vi "Update Target Value.vi"(11 "Target Info":T1(array[cluster])) -> (3 "Was target seen?":bool)   [LabVIEW 2012]
uses:
  Target Datum.ctl
  Robot Global Data.vi
panel:
  in  "Bottom dividing line":dbl
  in  "Top dividing line":dbl
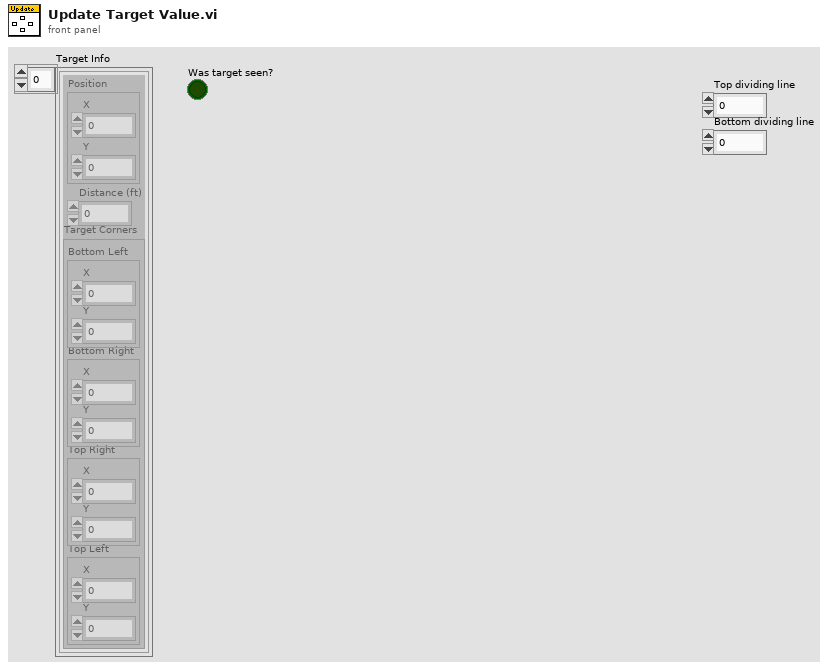
[diagram p1: front panel]
types:
  T1 = cluster{"Position":cluster{"X":dbl, "Y":dbl}, "Distance (ft)":dbl, "Target Corners":cluster{"Bottom Left":cluster{"X":dbl, "Y":dbl}, "Bottom Right":cluster{"X":dbl, "Y":dbl}, "Top Right":cluster{"X":dbl, "Y":dbl}, "Top Left":cluster{"X":dbl, "Y":dbl}}}[]
  T2 = typedef "Target Datum.ctl" = cluster{"Position":cluster{"X":dbl, "Y":dbl}, "Distance (ft)":dbl, "Target Corners":cluster{"Bottom Left":cluster{"X":dbl, "Y":dbl}, "Bottom Right":cluster{"X":dbl, "Y":dbl}, "Top Right":cluster{"X":dbl, "Y":dbl}, "Top Left":cluster{"X":dbl, "Y":dbl}}}
  T3 = cluster{"Left":T2, "Bottom":T2, "Right":T2, "Top":T2}
  T4 = cluster{"Position":cluster{"X":dbl, "Y":dbl}, "Distance (ft)":dbl, "Target Corners":cluster{"Bottom Left":cluster{"X":dbl, "Y":dbl}, "Bottom Right":cluster{"X":dbl, "Y":dbl}, "Top Right":cluster{"X":dbl, "Y":dbl}, "Top Left":cluster{"X":dbl, "Y":dbl}}}
  T5 = typedef "BasketType.ctl" = enum16{"Left", "Bottom", "Right", "Top"}
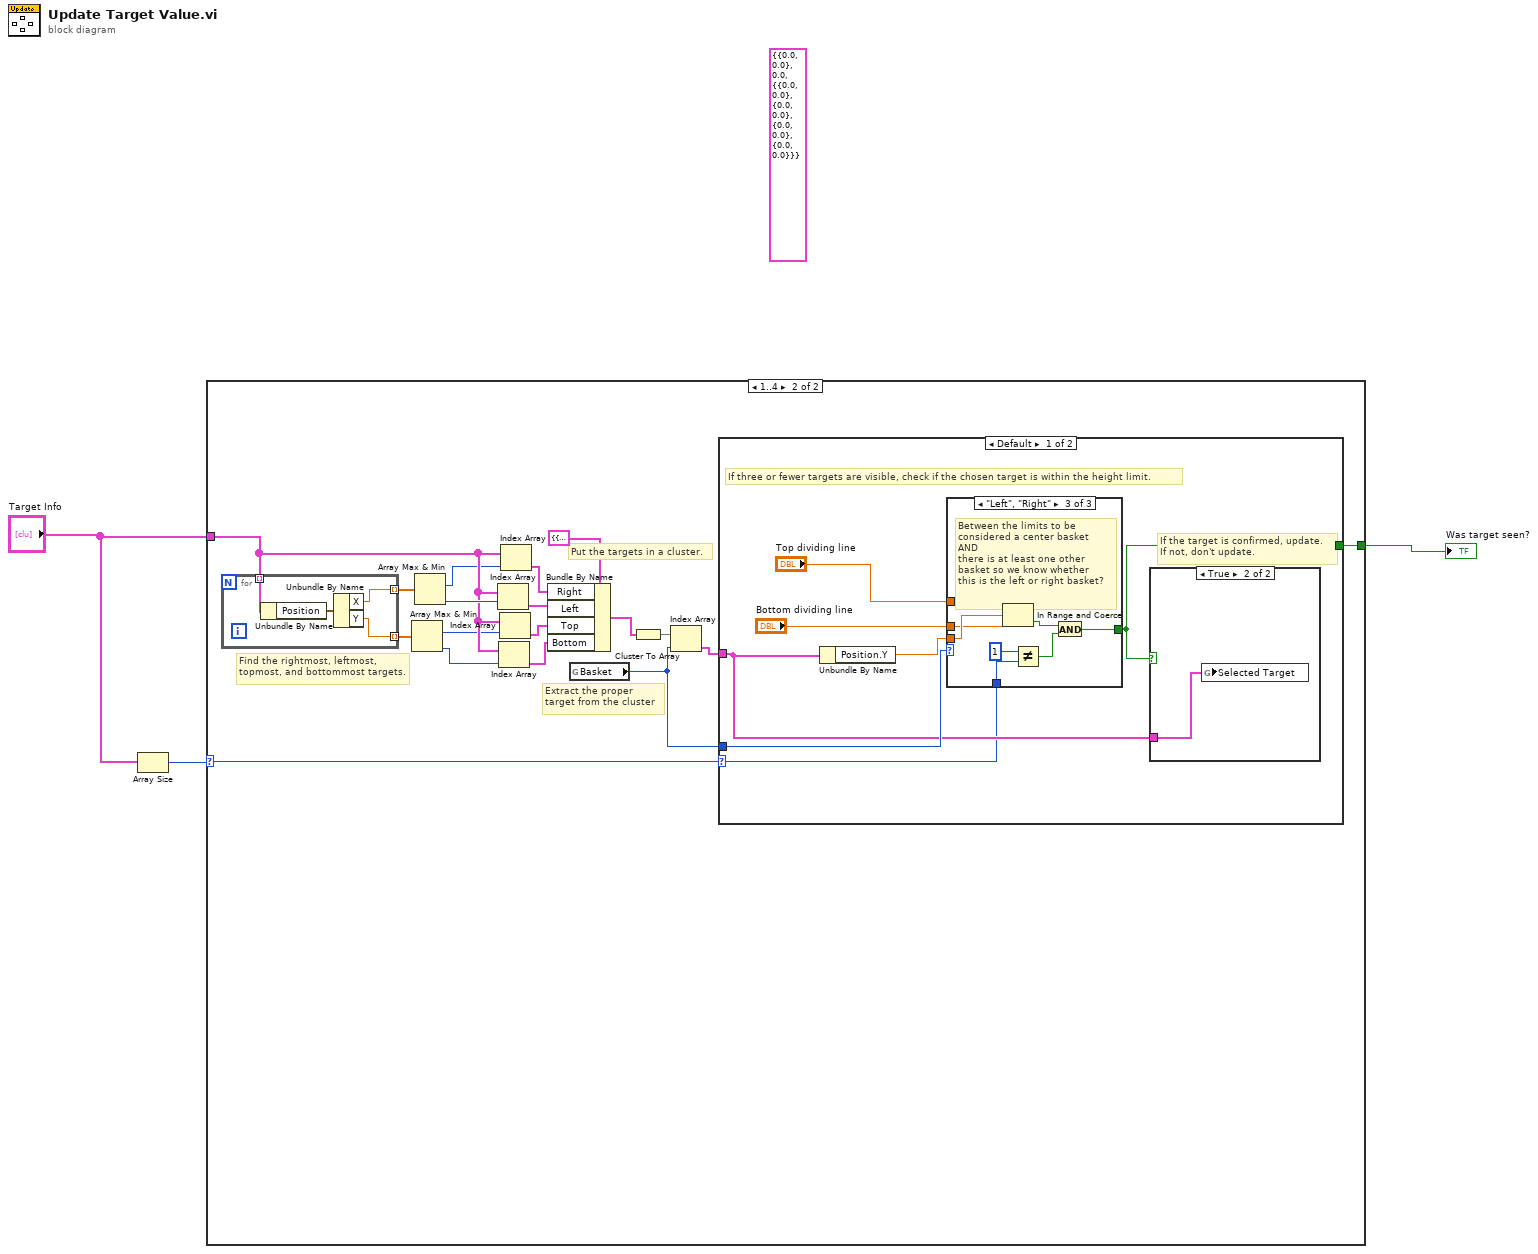
[diagram p0: block diagram]
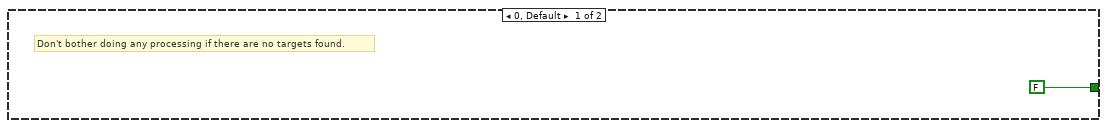
[diagram p2: hidden frame]
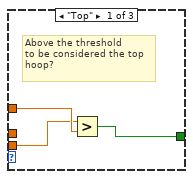
[diagram p4: hidden frame]
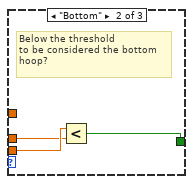
[diagram p5: hidden frame]
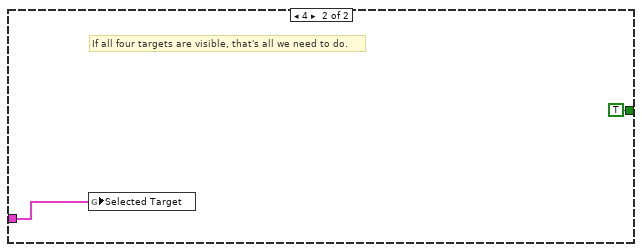
[diagram p6: hidden frame]
diagram:
  (unwired) T2 {"Position"={"X"=0.0, "Y"=0.0}, "Distance (ft)"=0.0, "Target Corners"={"Bottom Left"={"X"=0.0, "Y"=0.0}, "Bottom Right"={"X"=0.0, "Y"=0.0}, "Top Right"={"X"=0.0, "Y"=0.0}, "Top Left"={"X"=0.0, "Y"=0.0}}}
  n1 = Array Size(array="Target Info") -> (size(s)=w3:i32)
  n2 = case shown="1..4" w3 {
    selector: w3 -> [_ w6]
    tunnel: "Target Info" -> [_ w18]
    tunnel: [FALSE w5] -> w1
    frame 0, Default {
      # "Don't bother doing any processing if there are no targets found."
    }
    frame 1..4 {
      # "Extract the proper\ntarget from the cluster"
      # "Put the targets in a cluster."
      # "Find the rightmost, leftmost, topmost, and bottommost targets."
      n3 = for {
        tunnel: w18 -> [w50] mode=indexing
        tunnel: [w48] -> w20 mode=indexing
        tunnel: [w47] -> w22 mode=indexing
        n4 = Unbundle By Name(w50) -> ("Position"=w49:cluster{"X":dbl, "Y":dbl})
        n5 = Unbundle By Name(w49) -> ("X"=w48:dbl, "Y"=w47:dbl)
      }
      n6 = Array Max & Min(array=w22) -> (max index (indices)=w17:i32, min index (indices)=w21:i32)  [unwired: 2 out]
      n7 = Array Max & Min(array=w20) -> (max index (indices)=w16:i32, min index (indices)=w19:i32)  [unwired: 2 out]
      n8 = Index Array(array=w18, index=w19) -> (element=w13:T4)
      n9 = Index Array(array=w18, index=w21) -> (element=w11:T4)
      n10 = Index Array(array=w18, index=w17) -> (element=w12:T4)
      n11 = Index Array(array=w18, index=w16) -> (element=w14:T4)
      n12 = Bundle By Name(cluster=T3 {"Left"={"Position"={"X"=0.0, "Y"=0.0}, "Distance (ft)"=0.0, "Target Corners"={"Bottom Left"={"X"=0.0, "Y"=0.0}, "Bottom Right"={"X"=0.0, "Y"=0.0}, "Top Right"={"X"=0.0, "Y"=0.0}, "Top Left"={"X"=0.0, "Y"=0.0}}}, "Bottom"={"Position"={"X"=0.0, "Y"=0.0}, "Distance (ft)"=-1.0, "Target Corners"={"Bottom Left"={"X"=0.0, "Y"=0.0}, "Bottom Right"={"X"=0.0, "Y"=0.0}, "Top Right"={"X"=0.0, "Y"=0.0}, "Top Left"={"X"=0.0, "Y"=0.0}}}, "Right"={"Position"={"X"=0.0, "Y"=0.0}, "Distance (ft)"=0.0, "Target Corners"={"Bottom Left"={"X"=0.0, "Y"=0.0}, "Bottom Right"={"X"=0.0, "Y"=0.0}, "Top Right"={"X"=0.0, "Y"=0.0}, "Top Left"={"X"=0.0, "Y"=0.0}}}, "Top"={"Position"={"X"=0.0, "Y"=0.0}, "Distance (ft)"=0.0, "Target Corners"={"Bottom Left"={"X"=0.0, "Y"=0.0}, "Bottom Right"={"X"=0.0, "Y"=0.0}, "Top Right"={"X"=0.0, "Y"=0.0}, "Top Left"={"X"=0.0, "Y"=0.0}}}} ("Cluster"), "Right"=w14, "Left"=w13, "Top"=w12, "Bottom"=w11) -> (w10:T3)
      n13 = global read "Robot Global Data.vi" "Basket"() -> (w7:T5)
      n14 = Cluster To Array(cluster=w10) -> (array=w8:T2[])
      n15 = Index Array(array=w8, index=w7) -> (element=w9:T2)
      n16 = case shown="Default" w6 {
        selector: w6 -> [w24 _]
        tunnel: w9 -> [w25 w46]
        tunnel: w7 -> [w29 _]
        tunnel: [w23 TRUE] -> w5
        frame Default {
          # "If the target is confirmed, update.\nIf not, don't update."
          # "If three or fewer targets are visible, check if the chosen target is within the height limit."
          n17 = Unbundle By Name(w25) -> ("Position.Y"=w27:dbl)
          n18 = case shown="\"Left\", \"Right\"" w29 {
            tunnel: "Top dividing line" -> [w33 _ w44]
            tunnel: w27 -> [w32 w36 w43]
            tunnel: [w31 w35 w39] -> w23
            tunnel: "Bottom dividing line" -> [_ w34 w42]
            tunnel: w24 -> [_ _ w41]
            frame "Top" {
              # "Above the threshold\nto be considered the top\nhoop?"
              n19 = Greater?(x=w32, y=w33) -> (0:w31:bool)
            }
            frame "Bottom" {
              # "Below the threshold\nto be considered the bottom\nhoop?"
              n20 = Less?(x=w36, y=w34) -> (x < y?=w35:bool)
            }
            frame "Left", "Right" {
              # "Between the limits to be\nconsidered a center basket\nAND\nthere is at least one other\nbasket so we know whether\nthis is the left or right basket?"
              n21 = In Range and Coerce(upper limit=w44, x=w43, lower limit=w42) -> (In Range?=w38:bool)  [unwired: 1 out]
              n22 = Not Equal?(x=1, y=w41) -> (x != y?=w37:bool)
              n23 = And(x=w38, y=w37) -> (x .and. y?=w39:bool)
            }
          }
          n24 = case shown="True" w23 {
            tunnel: w25 -> [_ w30]
            frame False {
            }
            frame True {
              n25 = global write "Robot Global Data.vi" "Selected Target"(w30) -> ()
            }
          }
        }
        frame 4 {
          # "If all four targets are visible, that's all we need to do."
          n26 = global write "Robot Global Data.vi" "Selected Target"(w46) -> ()
        }
      }
    }
  }
  "Was target seen?" <- w1
